vi "kvCanRead.vi"(6 "error in (no error)":errorcluster, 8 "Channel Handle (input only)":i32) -> (0 "Message Data":u8[](array[numeric]), 1 "error out":errorcluster, 2 "Message Timestamp":u32, 3 "Message Flags":u32, 4 "Channel Handle (output only)":i32, 5 "Message Id":i32)   [LabVIEW 2022 SP3]
doc: "Reads a message from the receive buffer. If no message is available, the function returns immediately with return code canERR_NOMSG."
uses:
  canlib32.dll
panel:
  # "8"
  # "16"
  # "24"
  # "32"
  # "40"
  # "48"
  # "56"
  # "64"
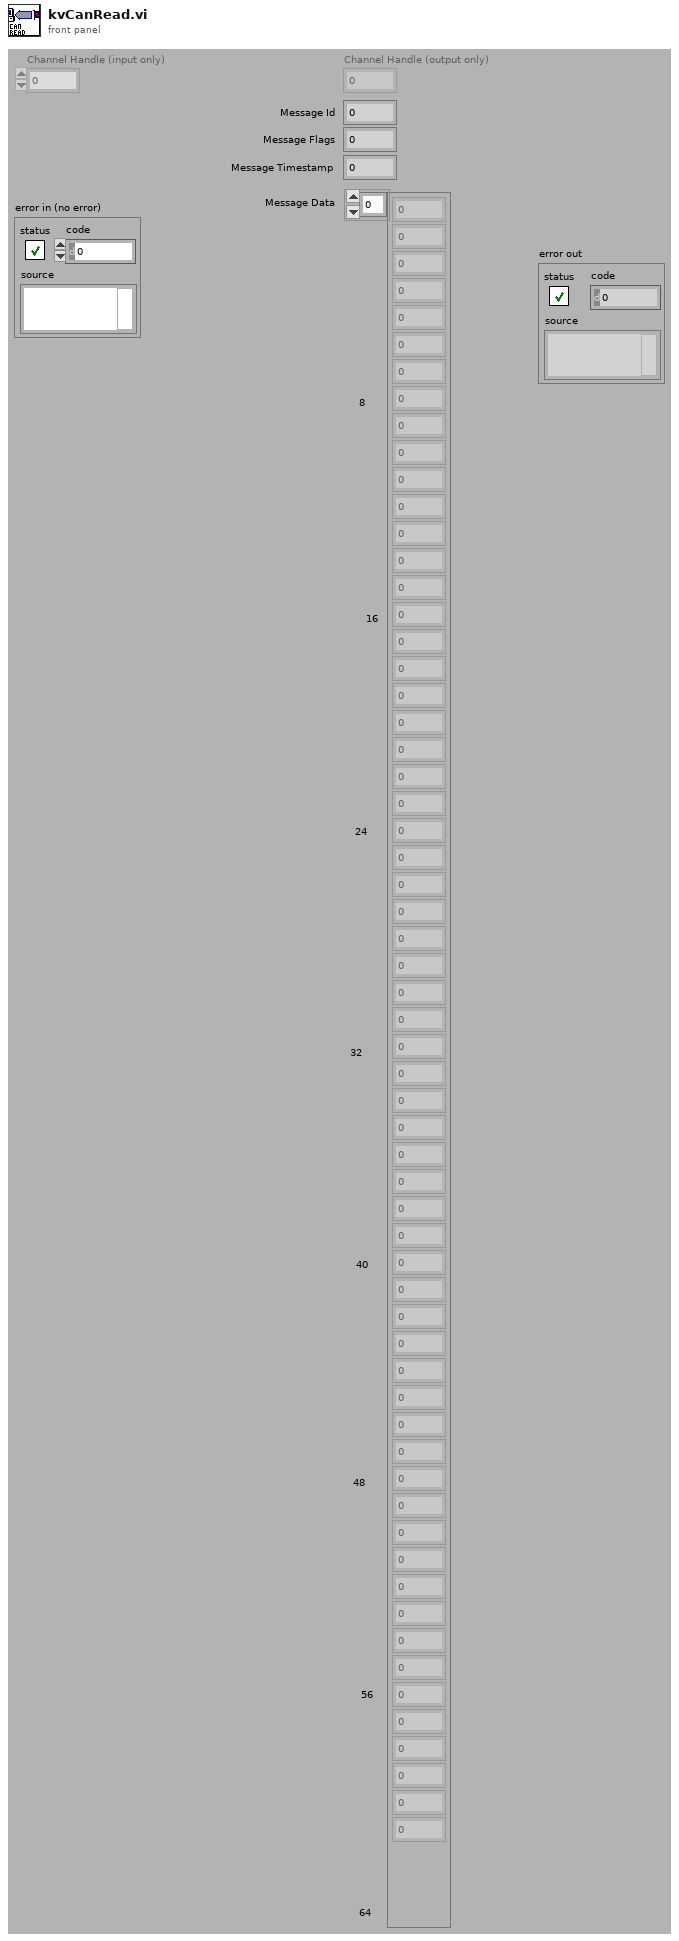
[diagram p1: front panel]
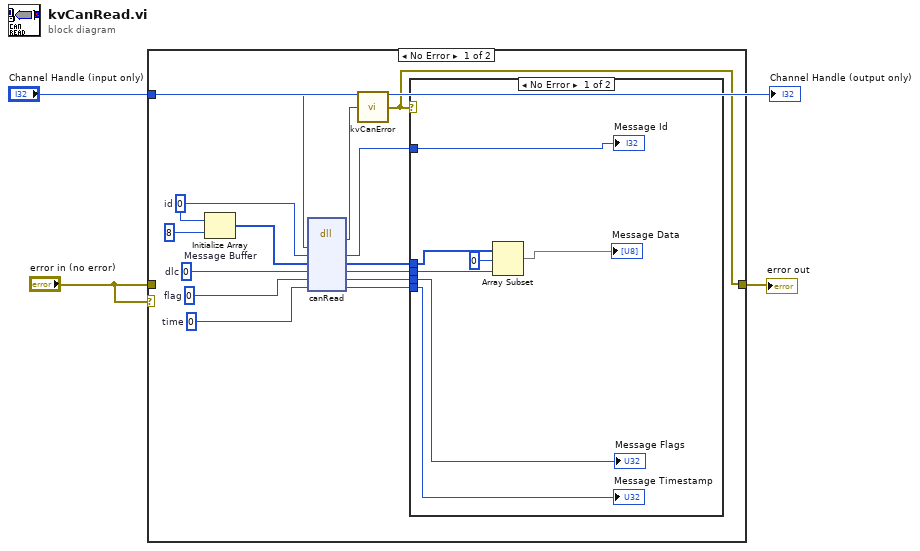
[diagram p0: block diagram]
diagram:
  n1 = case shown="No Error" "error in (no error)" {
    tunnel: [w4 w25] -> w2
    tunnel: "error in (no error)" -> [_ w25]
    tunnel: "Channel Handle (input only)" -> [w17 _]
    frame No Error {
      w13 = 0  # time
      w12 = 0  # flag
      w11 = 0  # dlc
      w16 = 0  # id
      n2 = Initialize Array "Message Buffer"(w16, 8) -> (w14:i32[])
      n3 = dll-call lib="canlib32.dll" fn="canRead"("handle"=w17, "id"=w16, "msg"=w14, "dlc"=w11, "flag"=w12, "time"=w13) -> (w10:i32, "id"=w9:i32, "msg"=w5:u8[], "dlc"=w6:u32, "flag"=w7:u32, "time"=w8:u32)  [unwired: 4 in, 2 out]
      n4 = call "kvCanError.vi"("error code"=w10) -> ("error out"=w4:errorcluster)
      n5 = case shown="No Error" w4 {
        tunnel: w9 -> [w24 _]
        tunnel: w8 -> [w23 _]
        tunnel: w7 -> [w22 _]
        tunnel: w6 -> [w18 _]
        tunnel: w5 -> [w21 _]
        frame No Error {
          n6 = Array Subset(array=w21, index=u32 0, length=w18) -> (→"Message Data":u8[])
          "Message Timestamp" <- w23
          "Message Flags" <- w22
          "Message Id" <- w24
        }
        frame Error {
        }
      }
    }
    frame Error {
    }
  }
  "error out" <- w2
  "Channel Handle (output only)" <- "Channel Handle (input only)"
